vi "CRYTS Tree Fresh Lib.vi"(0 "sOption":string, 5 "Steps":T2[](array[typedef]) {"Repeat State Array"."Start" format="%#_5g"; "Y dB ref" format="%.1f"; "Y data" items=["dB", "Lin"]; "Start" format="%#_5g"}, 7 "EditStepNo":u16) -> (4 "Tree Items":T1(array[cluster]), 6 "Edit Step Index":i32)   [LabVIEW 2013]
uses:
  CRYSystem/Typedef Control/CRYStep.ctl
panel:
  in  "Temp No":i32
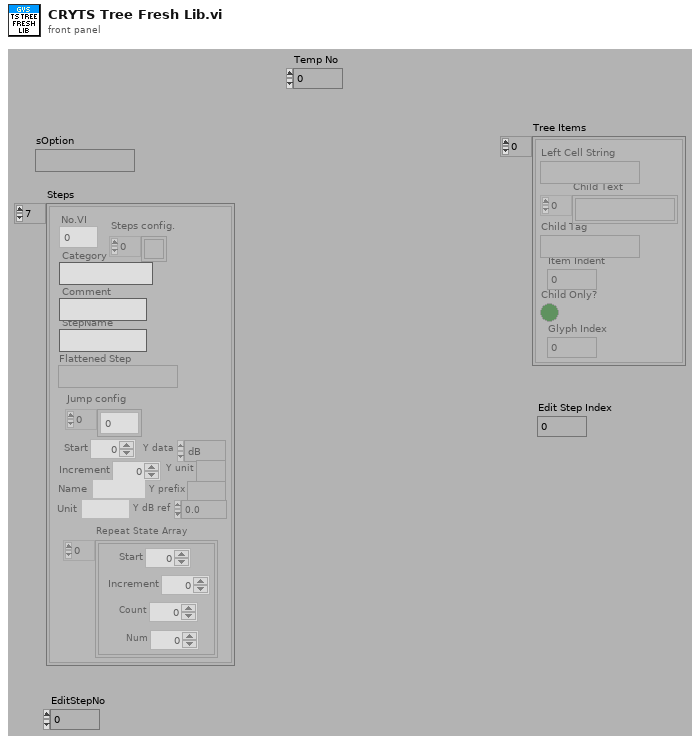
[diagram p1: front panel]
types:
  T1 = cluster{"Left Cell String":string, "Child Text":string[], "Child Tag":string, "Item Indent":i32, "Child Only?":bool, "Glyph Index":i32}[]
  T2 = typedef "CRYStep.ctl" = cluster{"No.VI":i32, "Category":string, "StepName":string, "Seq setup flattened":string, "Comment":string, "Steps config.":bool[], "Jump config":i32[], "Start":dbl, "Increment":dbl, "Name":string, "Unit":string, "Y data":u16, "Y prefix":string, "Y dB ref":dbl, "Y unit":string, "Repeat State Array":cluster{"Start":dbl, "Increment":dbl, "Count":i32, "Num":i32}[]}
  T3 = cluster{"Left Cell String":string, "Child Text":string[], "Child Tag":string, "Item Indent":i32, "Child Only?":bool, "Glyph Index":i32}
  T4 = cluster{"Start":dbl, "Increment":dbl, "Count":i32, "Num":i32}[]
  T5 = typedef "CRYStart Cluster.ctl" = cluster{"SequenceName":string, "Preload Stimulus":bool, "CloseOpenedDisplay":bool, "ClearMeasuredData":bool, "UpdateDisplayDuringRun":bool, "DisplayForConfirmation":bool, "HaltOnFail":bool, "UseSameHardware":bool, "UseSameCalibration":bool}
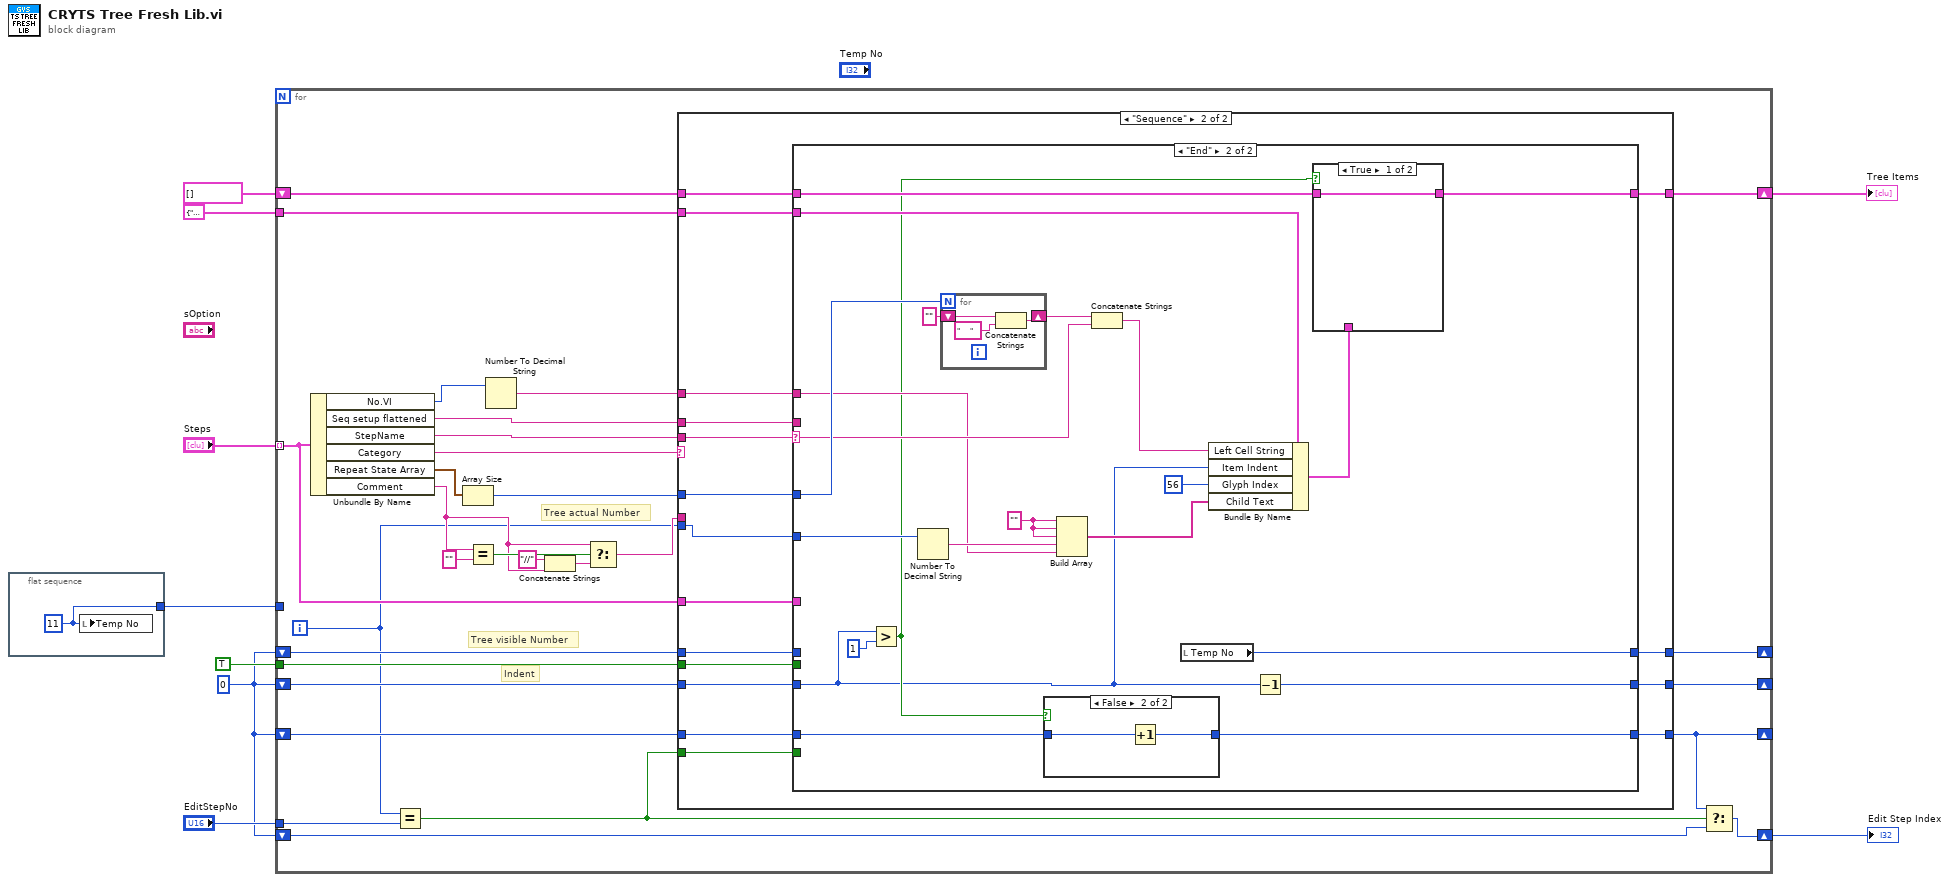
[diagram p0: block diagram]
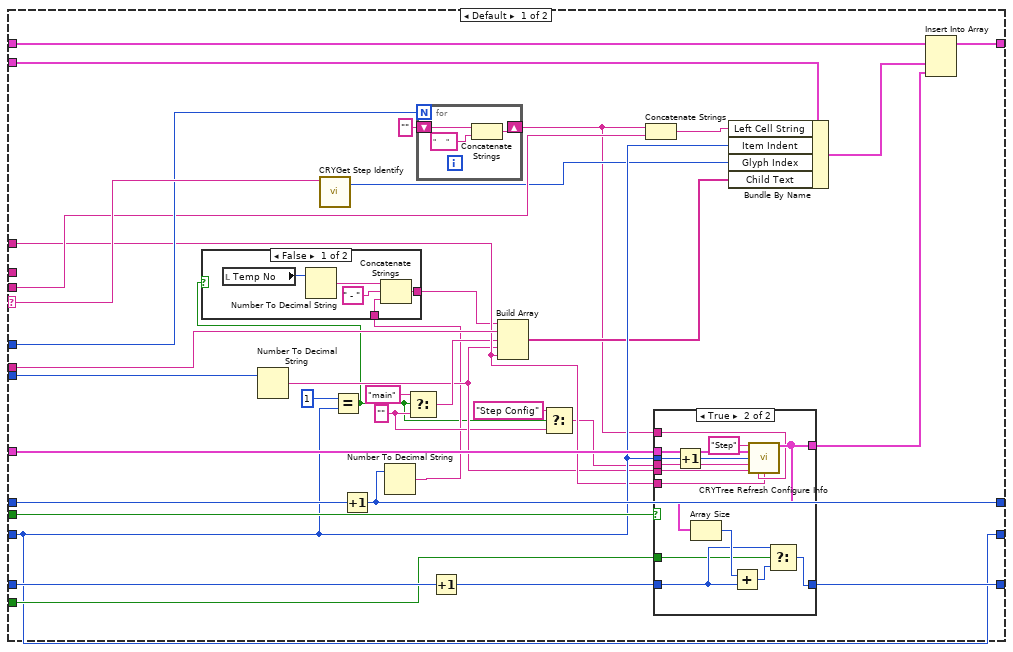
[diagram p2: hidden frame]
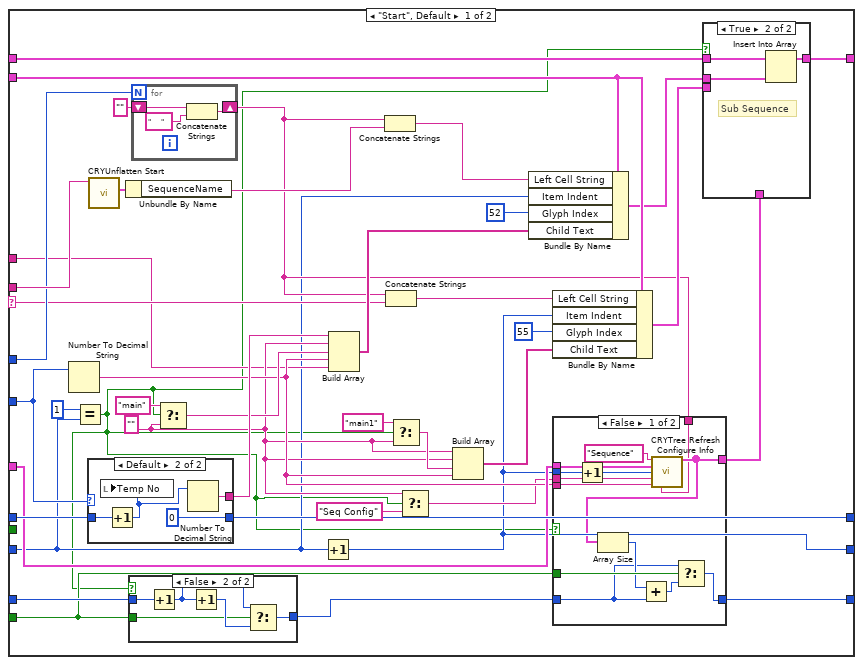
[diagram p5: hidden frame]
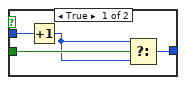
[diagram p6: hidden frame]
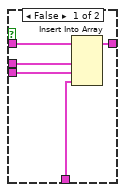
[diagram p7: hidden frame]
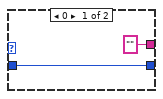
[diagram p9: hidden frame]
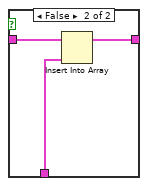
[diagram p11: hidden frame]
diagram:
  w2 = 0 ("Glyph Index")
  n1 = flat-sequence {
    tunnel: [w10] -> w1
    frame #0 {
      w10 = 11 ("Temp No")
      n2 = local write "Temp No"(w10) -> ()
    }
  }
  n3 = for {
    tunnel: T3 {"Left Cell String"="", "Child Text"=[], "Child Tag"="", "Item Indent"=0, "Child Only?"=FALSE, "Glyph Index"=0} ("Item") -> [w39]
    shift-right: [w37] -> w9
    shift-left: T1 [] -> [w38]
    shift-right: [w36] -> _
    shift-left: w2 -> [w35]
    tunnel: "EditStepNo" -> [w33]
    shift-right: [w30] -> _
    shift-left: w2 -> [w34]
    shift-right: [w31] -> w4
    shift-left: w2 -> [w32]
    shift-right: [w26] -> _
    shift-left: w2 -> [w27]
    tunnel: "Steps" -> [w16] mode=indexing
    tunnel: TRUE ("ConfigureShow") -> [w15]
    tunnel: w1 -> [_]
    i -> [w11]
    # "Tree actual Number"
    # "Tree visible Number"
    # "Indent"
    n4 = Unbundle By Name(w16) -> ("No.VI"=w13:i32, "Seq setup flattened"=w25:string, "StepName"=w24:string, "Category"=w23:string, "Repeat State Array"=w22:T4, "Comment"=w18:string)
    n5 = Equal?(x=w11, y=w33) -> (x = y?=w29:bool)
    n6 = Array Size(array=w22) -> (size(s)=w28:i32)
    n7 = Equal?(x=w18, y="") -> (x = y?=w20:bool)
    n8 = Number To Decimal String(number=w13) -> (decimal integer string=w12:string)  [unwired: 1 in]
    n9 = Concatenate Strings("//" ("string"), w18) -> (w17:string)
    n10 = Select(t=w18, s=w20, f=w17) -> (s? t:f=w19:string)
    n11 = case shown="\"Sequence\"" w23 {
      selector: w23 -> [w70 _]
      tunnel: w24 -> [w61 w115]
      tunnel: w39 -> [w72 w114]
      tunnel: w38 -> [w74 w113]
      tunnel: [w73 w112] -> w37
      tunnel: [w63 w111] -> w36
      tunnel: w35 -> [w63 w100]
      tunnel: w25 -> [_ w110]
      tunnel: w34 -> [w71 w101]
      tunnel: w11 -> [w58 w99]
      tunnel: [w66 w109] -> w30
      tunnel: w29 -> [w65 w108]
      tunnel: w28 -> [w62 w107]
      tunnel: w27 -> [w69 w106]
      tunnel: [w68 w105] -> w26
      tunnel: w19 -> [w60 _]
      tunnel: w16 -> [w67 w104]
      tunnel: w15 -> [w64 w103]
      tunnel: w12 -> [w59 w102]
      frame Default {
        w44 = "" ("decimal integer string")
        n12 = Number To Decimal String(number=w58) -> (decimal integer string=w51:string)  [unwired: 1 in]
        n13 = call "CRYGet Step Identify.vi"("Category Name In"=w70) -> ("Symbol Index"=w57:i32)  [unwired: 3 in, 7 out]
        n14 = Equal?(x=1 ("y"), y=w63) -> (x = y?=w40:bool)
        n15 = Increment(x=w69) -> (x+1=w68:i32)
        n16 = Number To Decimal String(number=w68) -> (decimal integer string=w42:string)  [unwired: 1 in]
        n17 = case shown="False" w40 {
          tunnel: w42 -> [w76 w80]
          tunnel: [w75 w80] -> w41
          frame False {
            n18 = local read "Temp No"() -> (w79:i32)
            n19 = Number To Decimal String(number=w79) -> (decimal integer string=w78:string)  [unwired: 1 in]
            n20 = Concatenate Strings(w78, " - " ("format string"), w76) -> (w75:string)
          }
          frame True {
          }
        }
        n21 = Select(t="main" ("decimal integer string"), s=w40, f=w44) -> (s? t:f=w53:string)
        n22 = for {
          N: w62 -> [_]
          shift-right: [w83] -> w45
          shift-left: "" ("decimal integer string") -> [w82]
          n23 = Concatenate Strings(w82, "     " ("decimal integer string")) -> (w83:string)
        }
        n24 = Increment(x=w71) -> (x+1=w48:i32)
        n25 = Build Array(w41, w60, w53, w51, w59) -> (w55:string[])
        n26 = Select(t="Step Config" ("SequenceName"), s=w40, f=w44) -> (s? t:f=w50:string)
        n27 = Concatenate Strings(w45, w61) -> (w46:string)
        n28 = case shown="True" w64 {
          tunnel: w63 -> [_ w97]
          tunnel: w67 -> [_ w96]
          tunnel: [_ w93] -> w43
          tunnel: w51 -> [_ w95]
          tunnel: w50 -> [_ w94]
          tunnel: w48 -> [w84 w91]
          tunnel: [w84 w88] -> w66
          tunnel: w65 -> [_ w90]
          tunnel: w45 -> [_ w86]
          tunnel: w59 -> [_ w85]
          frame False {
          }
          frame True {
            n29 = Increment(x=w97) -> (x+1=w87:i32)
            n30 = call "CRYTree Refresh Configure Info.vi"("sOption"="Step", "Step"=w96, "Item Indent"=w87, "Child3"=w94, "Child4"=w95, "SpaceStr"=w86, "Child5"=w85) -> ("Tree Items"=w93:T1)  [unwired: 8 in]
            n31 = Array Size(array=w93) -> (size(s)=w92:i32)
            n32 = Add(x=w92, y=w91) -> (x+y=w89:i32)
            n33 = Select(t=w91, s=w90, f=w89) -> (s? t:f=w88:i32)
          }
        }
        n34 = Bundle By Name(cluster=w72, "Left Cell String"=w46, "Item Indent"=w63, "Glyph Index"=w57, "Child Text"=w55) -> (w56:T3)
        n35 = Insert Into Array(array=w74, new element #1=w56, new element #2=w43) -> (w73:T1)  [unwired: 1 in]
      }
      frame "Sequence" {
        n36 = case shown="\"End\"" w115 {
          selector: w115 -> [w120 w203]
          tunnel: w100 -> [w117 w199]
          tunnel: w114 -> [w152 w217]
          tunnel: [w127 w213] -> w111
          tunnel: w113 -> [w154 w216]
          tunnel: [w153 w214] -> w112
          tunnel: w110 -> [w151 _]
          tunnel: w99 -> [w145 w209]
          tunnel: w101 -> [w148 w212]
          tunnel: [w129 w211] -> w109
          tunnel: w108 -> [w128 _]
          tunnel: w107 -> [w125 w206]
          tunnel: w106 -> [w144 _]
          tunnel: [w143 w197] -> w105
          tunnel: w104 -> [w137 _]
          tunnel: w103 -> [_ _]
          tunnel: w102 -> [w118 w201]
          frame "Start", Default {
            w119 = "" ("decimal integer string")
            n37 = Number To Decimal String(number=w145) -> (decimal integer string=w133:string)  [unwired: 1 in]
            n38 = Equal?(x=1 ("y"), y=w117) -> (x = y?=w116:bool)
            n39 = case shown="Default" w145 {
              tunnel: w144 -> [w192 w194]
              tunnel: [w192 0 ("Glyph Index")] -> w143
              tunnel: ["" w195] -> w142
              frame 0 {
              }
              frame Default {
                n40 = Increment(x=w194) -> (x+1=w193:i32)
                n41 = local write "Temp No"(w193) -> ()
                n42 = Number To Decimal String(number=w193) -> (decimal integer string=w195:string)  [unwired: 1 in]
              }
            }
            n43 = call "CRYUnflatten Start.vi"("Unflatten Sequence"=w151) -> ("Sequence Configure"=w150:T5)  [unwired: 8 in, 2 out]
            n44 = Unbundle By Name(w150) -> ("SequenceName"=w124:string)
            n45 = case shown="False" w116 {
              tunnel: w148 -> [w160 w165]
              tunnel: [w159 w162] -> w130
              tunnel: w128 -> [w158 w161]
              frame True {
                n46 = Increment(x=w160) -> (x+1=w157:i32)
                n47 = Select(t=w157, s=w158, f=w157) -> (s? t:f=w159:i32)
              }
              frame False {
                n48 = Increment(x=w165) -> (x+1=w163:i32)
                n49 = Increment(x=w163) -> (x+1=w164:i32)
                n50 = Select(t=w163, s=w161, f=w164) -> (s? t:f=w162:i32)
              }
            }
            n51 = for {
              N: w125 -> [_]
              shift-right: [w176] -> w121
              shift-left: "" ("decimal integer string") -> [w175]
              n52 = Concatenate Strings(w175, "     " ("decimal integer string")) -> (w176:string)
            }
            n53 = Select(t="main" ("decimal integer string"), s=w116, f=w119) -> (s? t:f=w141:string)
            n54 = Increment(x=w117) -> (x+1=w127:i32)
            n55 = Build Array(w142, w119, w141, w133, w118) -> (w149:string[])
            n56 = Concatenate Strings(w121, w124) -> (w123:string)
            n57 = Concatenate Strings(w121, w120) -> (w122:string)
            n58 = Select(t="main1" ("decimal integer string"), s=w116, f=w119) -> (s? t:f=w138:string)
            n59 = Select(t=w119, s=w116, f="Seq Config" ("SequenceName")) -> (s? t:f=w131:string)
            n60 = Build Array(w119, w119, w138, w133) -> (w140:string[])
            n61 = Bundle By Name(cluster=w152, "Left Cell String"=w123, "Item Indent"=w117, "Glyph Index"=52, "Child Text"=w149) -> (w136:T3)
            n62 = Bundle By Name(cluster=w152, "Left Cell String"=w122, "Item Indent"=w127, "Glyph Index"=55, "Child Text"=w140) -> (w135:T3)
            n63 = case shown="False" w116 {
              tunnel: w137 -> [w188 _]
              tunnel: [w184 _] -> w134
              tunnel: w127 -> [w187 _]
              tunnel: w133 -> [w186 _]
              tunnel: w131 -> [w185 _]
              tunnel: w130 -> [w180 w190]
              tunnel: [w179 w190] -> w129
              tunnel: w128 -> [w183 _]
              tunnel: w121 -> [w177 _]
              frame False {
                n64 = Increment(x=w187) -> (x+1=w178:i32)
                n65 = call "CRYTree Refresh Configure Info.vi"("sOption"="Sequence", "Step"=w188, "Item Indent"=w178, "Child3"=w185, "Child4"=w186, "SpaceStr"=w177) -> ("Tree Items"=w184:T1)  [unwired: 9 in]
                n66 = Array Size(array=w184) -> (size(s)=w182:i32)
                n67 = Add(x=w182, y=w180) -> (x+y=w181:i32)
                n68 = Select(t=w180, s=w183, f=w181) -> (s? t:f=w179:i32)
              }
              frame True {
                # "Sub Sequence"
              }
            }
            n69 = case shown="True" w116 {
              tunnel: w154 -> [w170 w173]
              tunnel: [w169 w172] -> w153
              tunnel: w136 -> [w168 w171]
              tunnel: w135 -> [w167 _]
              tunnel: w134 -> [w166 _]
              frame False {
                n70 = Insert Into Array(array=w170, new element #1=w168, new element #2=w167, new element #3=w166) -> (w169:T1)  [unwired: 1 in]
              }
              frame True {
                # "Sub Sequence"
                n71 = Insert Into Array(array=w173, new element=w171) -> (w172:T1)  [unwired: 1 in]
              }
            }
          }
          frame "End" {
            w207 = "" ("element")
            n72 = Greater?(x=w199, y=1) -> (0:w200:bool)
            n73 = Number To Decimal String(number=w209) -> (decimal integer string=w210:string)  [unwired: 1 in]
            n74 = for {
              N: w206 -> [_]
              shift-right: [w228] -> w204
              shift-left: "" ("decimal integer string") -> [w227]
              n75 = Concatenate Strings(w227, "     " ("decimal integer string")) -> (w228:string)
            }
            n76 = case shown="False" w200 {
              tunnel: w212 -> [w219 w221]
              tunnel: [w219 w220] -> w211
              frame True {
              }
              frame False {
                n77 = Increment(x=w221) -> (x+1=w220:i32)
              }
            }
            n78 = Build Array(w207, w207, w207, w210, w201) -> (w208:string[])
            n79 = Concatenate Strings(w204, w203) -> (w202:string)
            n80 = local read "Temp No"() -> (w197:i32)
            n81 = Bundle By Name(cluster=w217, "Left Cell String"=w202, "Item Indent"=w199, "Glyph Index"=56, "Child Text"=w208) -> (w215:T3)
            n82 = Decrement(x=w199) -> (x-1=w213:i32)
            n83 = case shown="True" w200 {
              tunnel: w216 -> [w222 w225]
              tunnel: w215 -> [_ w224]
              tunnel: [w222 w223] -> w214
              frame True {
              }
              frame False {
                n84 = Insert Into Array(array=w225, new element=w224) -> (w223:T1)  [unwired: 1 in]
              }
            }
          }
        }
      }
    }
    n85 = Select(t=w30, s=w29, f=w32) -> (s? t:f=w31:i32)
  }
  "Tree Items" <- w9
  "Edit Step Index" <- w4
